vi "Request Data JSON.vi"(8 "error in (no error)":errorcluster, 11 "SetCurrentProfile in":refnum<class "RemoveProfile.lvclass">) -> (0 "error out":errorcluster, 2 "Request Data JSON":string, 3 "SetCurrentProfile out":refnum<class "RemoveProfile.lvclass">)   [LabVIEW 2020, in "obs-websocket.lvlib" / "RemoveProfile.lvclass"]
uses:
  RemoveProfile.lvclass
  RemoveProfile.lvclass/RemoveProfile.ctl
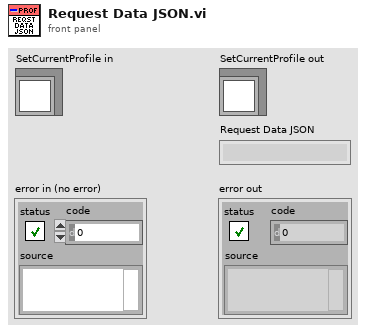
[diagram p1: front panel]
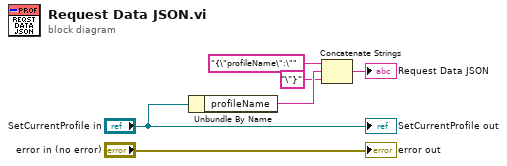
[diagram p0: block diagram]
diagram:
  n1 = Unbundle By Name("SetCurrentProfile in") -> ("profileName"=w4:string)
  n2 = Concatenate Strings("{\"profileName\":\"" ("string"), w4, "\"}" ("string")) -> (→"Request Data JSON":string)
  "error out" <- "error in (no error)"
  "SetCurrentProfile out" <- "SetCurrentProfile in"
